vi "Mark Persisted.vi"(10 "Entity ID":T1, 11 "Entity in":refnum<class "Entity.lvclass">) -> (3 "Entity out":refnum<class "Entity.lvclass">)   [LabVIEW 2020, in "Conditu2.lvlib" / "Entity.lvclass"]
uses:
  Entity.lvclass
  Entity ID.ctl
  Entity.lvclass/Entity.ctl
  Columns/ID/ID.lvclass/ID.ctl
  Entity State.ctl
  Columns/ID/Set.vi
  Conditu2.lvlib
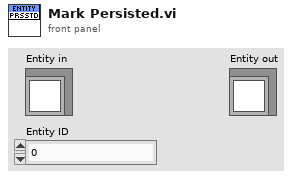
[diagram p1: front panel]
types:
  T1 = typedef "Conditu2.lvlib/Entity ID.ctl" = i64
  T2 = typedef "Conditu2.lvlib/Entity State.ctl" = enum16{"New", "Managed", "Detached", "Removed"}
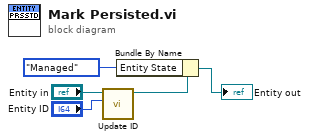
[diagram p0: block diagram]
diagram:
  n1 = call "Update ID.vi"("Entity ID"="Entity ID", "Entity in"="Entity in") -> ("Entity out"=w3:refnum<class "Entity.lvclass">)  [unwired: 9 in]
  n2 = Bundle By Name(cluster=w3, "Entity State"=Entity_State."Managed") -> (→"Entity out":refnum<class "Entity.lvclass">)
